vi "PicoScopeospaSettings.vi"(0 "handle in":i16=16384, 1 "Device Info":T3={"PICO_DRIVER_VERSION"="", "PICO_USB_VERSION"="", "PICO_HARDWARE_VERSION"="", "PICO_VARIANT_INFO"="", "PICO_BATCH_AND_SERIAL"="", "PICO_CAL_DATE"="", "PICO_KERNEL_VERSION"="", "PICO_DIGITAL_HARDWARE_VERSION"="", "PICO_ANALOGUE_HARDWARE_VERSION"="", "PICO_FIRMWARE_VERSION_1"="", "PICO_FIRMWARE_VERSION_2"="", "PICO_IPP_VERSION"="", "PICO_DRIVER_PATH"="", "PICO_FIRMWARE_VERSION_3"="", "PICO_FRONT_PANEL_FIRMWARE_VERSION"="", "Number of Channels"=0, "MSO"=TRUE}, 2 "Channels":T2={"Channel A Settings "={"Enabled"=FALSE, "Coupling"=1, "Range"=8, "Analogue Offset"=0.0, "BandWidth"=0, "PROBE_RANGE_INFO"=0}, "Channel B Settings "={"Enabled"=FALSE, "Coupling"=1, "Range"=8, "Analogue Offset"=0.0, "BandWidth"=0, "PROBE_RANGE_INFO"=0}, "Channel C Settings "={"Enabled"=FALSE, "Coupling"=1, "Range"=8, "Analogue Offset"=0.0, "BandWidth"=0, "PROBE_RANGE_INFO"=0}, "Channel D Settings "={"Enabled"=FALSE, "Coupling"=1, "Range"=8, "Analogue Offset"=0.0, "BandWidth"=0, "PROBE_RANGE_INFO"=0}, "Channel E Settings "={"Enabled"=FALSE, "Coupling"=50, "Range"=5, "Analogue Offset"=0.0, "BandWidth"=0, "PROBE_RANGE_INFO"=0}, "Channel F Settings "={"Enabled"=FALSE, "Coupling"=50, "Range"=5, "Analogue Offset"=0.0, "BandWidth"=0, "PROBE_RANGE_INFO"=0}, "Channel G Settings "={"Enabled"=FALSE, "Coupling"=50, "Range"=5, "Analogue Offset"=0.0, "BandWidth"=0, "PROBE_RANGE_INFO"=0}, "Channel H Settings "={"Enabled"=FALSE, "Coupling"=50, "Range"=5, "Analogue Offset"=0.0, "BandWidth"=0, "PROBE_RANGE_INFO"=0}} {"Channel H Settings"."PROBE_RANGE_INFO" items=["PROBE_NONE_NV"=0, "X1_PROBE_NV"=1, "X10_PROBE_NV"=10]; "Channel H Settings"."BandWidth" items=["Full"=0, "100kHz"=100000, "20kHz"=200000, "1MHz"=1000000, "20MHz"=20000000, "25MHz"=25000000, "50MHz"=50000000, "200MHz"=200000000, "250MHz"=250000000, "500MHz"=500000000]; "Channel H Settings"."Range" items=["10mV"=0, "20mV"=1, "50mV"=2, "100mV"=3, "200mV"=4, "500mV"=5, "1V"=6, "2V"=7, "5V"=8, "10V"=9, "20V"=10, "50V"=11, "100V"=12, "200V"=13, "x10_Probe_100mV"=32, "x10_Probe_200mV"=33, "x10_Probe_500mV"=34, "x10_Probe_1V"=35, "x10_Probe_2V"=36, "x10_Probe_5V"=37, "x10_Probe_10V"=38, "x10_Probe_20V"=39, "x10_Probe_50V"=40, "x10_Probe_100V"=41, "x10_Probe_200V"=42, "x10_Probe_500V"=43, "CURRENT_CLAMP_60A_2A"=10500, "CURRENT_CLAMP_60A_5A"=10501, "CURRENT_CLAMP_60A_10A"=10502, "CURRENT_CLAMP_60A_20A"=10503, "CURRENT_CLAMP_60A_50A"=10504, "CURRENT_CLAMP_60A_60A"=10505, "CURRENT_CLAMP_60A_V2_0_5A"=10600, "CURRENT_CLAMP_60A_V2_1A"=10601, "CURRENT_CLAMP_60A_V2_2A"=10602, "CURRENT_CLAMP_60A_V2_5A"=10603, "CURRENT_CLAMP_60A_V2_10A"=10604, "CURRENT_CLAMP_60A_V2_20A"=10605, "CURRENT_CLAMP_60A_V2_50A"=10606, "CURRENT_CLAMP_60A_V2_60A"=10607, "RESISTANCE_LEAD_NEG5_TO_20OHM"=7000, "RESISTANCE_LEAD_NEG50_TO_200OHM"=7001, "RESISTANCE_LEAD_NEG500_TO_2KOHM"=7002, "RESISTANCE_LEAD_NEG5K_TO_20KOHM"=7003, "RESISTANCE_LEAD_NEG50K_TO_LEAD_200KOHM"=7004, "RESISTANCE_LEAD_NEG500K_TO_LEAD_2MOHM"=7005, "RESISTANCE_LEAD_DIODE_TEST"=7006, "HT_NEG3_TO_5KV"=8950, "HT_NEG3_TO_10KV"=8951, "HT_NEG5_TO_20KV"=8952, "HT_NEG5_TO_50KV"=8953, "HT_NEG5_TO_100KV"=8954, "HT_NEG3_TO_5KV_INVERTED"=8955, "HT_NEG3_TO_10KV_INVERTED"=8956, "HT_NEG5_TO_20KV_INVERTED"=8957, "HT_NEG5_TO_50KV_INVERTED"=8958, "HT_NEG5_TO_100KV_INVERTED"=8959, "TEMPERATURE_NEG50_TO_150DEGC"=9000, "PRESSURE_SENSOR_-100k-150k_PASCALS"=9100, "PRESSURE_SENSOR_-100k_TO_400k_PASCALS"=9101, "PRESSURE_SENSOR_-200k_TO_800k_PASCALS"=9102, "PRESSURE_SENSOR_-400k_TO_1600k_PASCALS"=9103, "PRESSURE_SENSOR_-400k_TO_3400k_PASCALS"=9104, "PRESSURE_SENSOR_-150k_TO_1350k_PASCALS"=9105]; "Channel H Settings"."Coupling" items=["AC"=0, "DC 1M Ohm"=1, "DC 50 Ohm"=50]; "Channel G Settings"."PROBE_RANGE_INFO" items=["PROBE_NONE_NV"=0, "X1_PROBE_NV"=1, "X10_PROBE_NV"=10]; "Channel G Settings"."BandWidth" items=["Full"=0, "100kHz"=100000, "20kHz"=200000, "1MHz"=1000000, "20MHz"=20000000, "25MHz"=25000000, "50MHz"=50000000, "200MHz"=200000000, "250MHz"=250000000, "500MHz"=500000000]; "Channel G Settings"."Range" items=["10mV"=0, "20mV"=1, "50mV"=2, "100mV"=3, "200mV"=4, "500mV"=5, "1V"=6, "2V"=7, "5V"=8, "10V"=9, "20V"=10, "50V"=11, "100V"=12, "200V"=13, "x10_Probe_100mV"=32, "x10_Probe_200mV"=33, "x10_Probe_500mV"=34, "x10_Probe_1V"=35, "x10_Probe_2V"=36, "x10_Probe_5V"=37, "x10_Probe_10V"=38, "x10_Probe_20V"=39, "x10_Probe_50V"=40, "x10_Probe_100V"=41, "x10_Probe_200V"=42, "x10_Probe_500V"=43, "CURRENT_CLAMP_60A_2A"=10500, "CURRENT_CLAMP_60A_5A"=10501, "CURRENT_CLAMP_60A_10A"=10502, "CURRENT_CLAMP_60A_20A"=10503, "CURRENT_CLAMP_60A_50A"=10504, "CURRENT_CLAMP_60A_60A"=10505, "CURRENT_CLAMP_60A_V2_0_5A"=10600, "CURRENT_CLAMP_60A_V2_1A"=10601, "CURRENT_CLAMP_60A_V2_2A"=10602, "CURRENT_CLAMP_60A_V2_5A"=10603, "CURRENT_CLAMP_60A_V2_10A"=10604, "CURRENT_CLAMP_60A_V2_20A"=10605, "CURRENT_CLAMP_60A_V2_50A"=10606, "CURRENT_CLAMP_60A_V2_60A"=10607, "RESISTANCE_LEAD_NEG5_TO_20OHM"=7000, "RESISTANCE_LEAD_NEG50_TO_200OHM"=7001, "RESISTANCE_LEAD_NEG500_TO_2KOHM"=7002, "RESISTANCE_LEAD_NEG5K_TO_20KOHM"=7003, "RESISTANCE_LEAD_NEG50K_TO_LEAD_200KOHM"=7004, "RESISTANCE_LEAD_NEG500K_TO_LEAD_2MOHM"=7005, "RESISTANCE_LEAD_DIODE_TEST"=7006, "HT_NEG3_TO_5KV"=8950, "HT_NEG3_TO_10KV"=8951, "HT_NEG5_TO_20KV"=8952, "HT_NEG5_TO_50KV"=8953, "HT_NEG5_TO_100KV"=8954, "HT_NEG3_TO_5KV_INVERTED"=8955, "HT_NEG3_TO_10KV_INVERTED"=8956, "HT_NEG5_TO_20KV_INVERTED"=8957, "HT_NEG5_TO_50KV_INVERTED"=8958, "HT_NEG5_TO_100KV_INVERTED"=8959, "TEMPERATURE_NEG50_TO_150DEGC"=9000, "PRESSURE_SENSOR_-100k-150k_PASCALS"=9100, "PRESSURE_SENSOR_-100k_TO_400k_PASCALS"=9101, "PRESSURE_SENSOR_-200k_TO_800k_PASCALS"=9102, "PRESSURE_SENSOR_-400k_TO_1600k_PASCALS"=9103, "PRESSURE_SENSOR_-400k_TO_3400k_PASCALS"=9104, "PRESSURE_SENSOR_-150k_TO_1350k_PASCALS"=9105]; "Channel G Settings"."Coupling" items=["AC"=0, "DC 1M Ohm"=1, "DC 50 Ohm"=50]; "Channel F Settings"."PROBE_RANGE_INFO" items=["PROBE_NONE_NV"=0, "X1_PROBE_NV"=1, "X10_PROBE_NV"=10]; "Channel F Settings"."BandWidth" items=["Full"=0, "100kHz"=100000, "20kHz"=200000, "1MHz"=1000000, "20MHz"=20000000, "25MHz"=25000000, "50MHz"=50000000, "200MHz"=200000000, "250MHz"=250000000, "500MHz"=500000000]; "Channel F Settings"."Range" items=["10mV"=0, "20mV"=1, "50mV"=2, "100mV"=3, "200mV"=4, "500mV"=5, "1V"=6, "2V"=7, "5V"=8, "10V"=9, "20V"=10, "50V"=11, "100V"=12, "200V"=13, "x10_Probe_100mV"=32, "x10_Probe_200mV"=33, "x10_Probe_500mV"=34, "x10_Probe_1V"=35, "x10_Probe_2V"=36, "x10_Probe_5V"=37, "x10_Probe_10V"=38, "x10_Probe_20V"=39, "x10_Probe_50V"=40, "x10_Probe_100V"=41, "x10_Probe_200V"=42, "x10_Probe_500V"=43, "CURRENT_CLAMP_60A_2A"=10500, "CURRENT_CLAMP_60A_5A"=10501, "CURRENT_CLAMP_60A_10A"=10502, "CURRENT_CLAMP_60A_20A"=10503, "CURRENT_CLAMP_60A_50A"=10504, "CURRENT_CLAMP_60A_60A"=10505, "CURRENT_CLAMP_60A_V2_0_5A"=10600, "CURRENT_CLAMP_60A_V2_1A"=10601, "CURRENT_CLAMP_60A_V2_2A"=10602, "CURRENT_CLAMP_60A_V2_5A"=10603, "CURRENT_CLAMP_60A_V2_10A"=10604, "CURRENT_CLAMP_60A_V2_20A"=10605, "CURRENT_CLAMP_60A_V2_50A"=10606, "CURRENT_CLAMP_60A_V2_60A"=10607, "RESISTANCE_LEAD_NEG5_TO_20OHM"=7000, "RESISTANCE_LEAD_NEG50_TO_200OHM"=7001, "RESISTANCE_LEAD_NEG500_TO_2KOHM"=7002, "RESISTANCE_LEAD_NEG5K_TO_20KOHM"=7003, "RESISTANCE_LEAD_NEG50K_TO_LEAD_200KOHM"=7004, "RESISTANCE_LEAD_NEG500K_TO_LEAD_2MOHM"=7005, "RESISTANCE_LEAD_DIODE_TEST"=7006, "HT_NEG3_TO_5KV"=8950, "HT_NEG3_TO_10KV"=8951, "HT_NEG5_TO_20KV"=8952, "HT_NEG5_TO_50KV"=8953, "HT_NEG5_TO_100KV"=8954, "HT_NEG3_TO_5KV_INVERTED"=8955, "HT_NEG3_TO_10KV_INVERTED"=8956, "HT_NEG5_TO_20KV_INVERTED"=8957, "HT_NEG5_TO_50KV_INVERTED"=8958, "HT_NEG5_TO_100KV_INVERTED"=8959, "TEMPERATURE_NEG50_TO_150DEGC"=9000, "PRESSURE_SENSOR_-100k-150k_PASCALS"=9100, "PRESSURE_SENSOR_-100k_TO_400k_PASCALS"=9101, "PRESSURE_SENSOR_-200k_TO_800k_PASCALS"=9102, "PRESSURE_SENSOR_-400k_TO_1600k_PASCALS"=9103, "PRESSURE_SENSOR_-400k_TO_3400k_PASCALS"=9104, "PRESSURE_SENSOR_-150k_TO_1350k_PASCALS"=9105]; "Channel F Settings"."Coupling" items=["AC"=0, "DC 1M Ohm"=1, "DC 50 Ohm"=50]; "Channel E Settings"."PROBE_RANGE_INFO" items=["PROBE_NONE_NV"=0, "X1_PROBE_NV"=1, "X10_PROBE_NV"=10]; "Channel E Settings"."BandWidth" items=["Full"=0, "100kHz"=100000, "20kHz"=200000, "1MHz"=1000000, "20MHz"=20000000, "25MHz"=25000000, "50MHz"=50000000, "200MHz"=200000000, "250MHz"=250000000, "500MHz"=500000000]; "Channel E Settings"."Range" items=["10mV"=0, "20mV"=1, "50mV"=2, "100mV"=3, "200mV"=4, "500mV"=5, "1V"=6, "2V"=7, "5V"=8, "10V"=9, "20V"=10, "50V"=11, "100V"=12, "200V"=13, "x10_Probe_100mV"=32, "x10_Probe_200mV"=33, "x10_Probe_500mV"=34, "x10_Probe_1V"=35, "x10_Probe_2V"=36, "x10_Probe_5V"=37, "x10_Probe_10V"=38, "x10_Probe_20V"=39, "x10_Probe_50V"=40, "x10_Probe_100V"=41, "x10_Probe_200V"=42, "x10_Probe_500V"=43, "CURRENT_CLAMP_60A_2A"=10500, "CURRENT_CLAMP_60A_5A"=10501, "CURRENT_CLAMP_60A_10A"=10502, "CURRENT_CLAMP_60A_20A"=10503, "CURRENT_CLAMP_60A_50A"=10504, "CURRENT_CLAMP_60A_60A"=10505, "CURRENT_CLAMP_60A_V2_0_5A"=10600, "CURRENT_CLAMP_60A_V2_1A"=10601, "CURRENT_CLAMP_60A_V2_2A"=10602, "CURRENT_CLAMP_60A_V2_5A"=10603, "CURRENT_CLAMP_60A_V2_10A"=10604, "CURRENT_CLAMP_60A_V2_20A"=10605, "CURRENT_CLAMP_60A_V2_50A"=10606, "CURRENT_CLAMP_60A_V2_60A"=10607, "RESISTANCE_LEAD_NEG5_TO_20OHM"=7000, "RESISTANCE_LEAD_NEG50_TO_200OHM"=7001, "RESISTANCE_LEAD_NEG500_TO_2KOHM"=7002, "RESISTANCE_LEAD_NEG5K_TO_20KOHM"=7003, "RESISTANCE_LEAD_NEG50K_TO_LEAD_200KOHM"=7004, "RESISTANCE_LEAD_NEG500K_TO_LEAD_2MOHM"=7005, "RESISTANCE_LEAD_DIODE_TEST"=7006, "HT_NEG3_TO_5KV"=8950, "HT_NEG3_TO_10KV"=8951, "HT_NEG5_TO_20KV"=8952, "HT_NEG5_TO_50KV"=8953, "HT_NEG5_TO_100KV"=8954, "HT_NEG3_TO_5KV_INVERTED"=8955, "HT_NEG3_TO_10KV_INVERTED"=8956, "HT_NEG5_TO_20KV_INVERTED"=8957, "HT_NEG5_TO_50KV_INVERTED"=8958, "HT_NEG5_TO_100KV_INVERTED"=8959, "TEMPERATURE_NEG50_TO_150DEGC"=9000, "PRESSURE_SENSOR_-100k-150k_PASCALS"=9100, "PRESSURE_SENSOR_-100k_TO_400k_PASCALS"=9101, "PRESSURE_SENSOR_-200k_TO_800k_PASCALS"=9102, "PRESSURE_SENSOR_-400k_TO_1600k_PASCALS"=9103, "PRESSURE_SENSOR_-400k_TO_3400k_PASCALS"=9104, "PRESSURE_SENSOR_-150k_TO_1350k_PASCALS"=9105]; "Channel E Settings"."Coupling" items=["AC"=0, "DC 1M Ohm"=1, "DC 50 Ohm"=50]; "Channel D Settings"."BandWidth" items=["Full"=0, "100kHz"=100000, "20kHz"=200000, "1MHz"=1000000, "20MHz"=20000000, "25MHz"=25000000, "50MHz"=50000000, "100MHz"=100000000, "200MHz"=200000000, "250MHz"=250000000, "350MHz"=350000000, "500MHz"=500000000]; "Channel D Settings"."PROBE_RANGE_INFO" items=["PROBE_NONE_NV"=0, "X1_PROBE_NV"=1, "X10_PROBE_NV"=10]; "Channel D Settings"."Range" items=["10mV", "20mV", "50mV", "100mV", "200mV", "500mV", "1V", "2V", "5V", "10V", "20V", "50V", "100V", "200V"]; "Channel D Settings"."Coupling" items=["AC"=0, "DC 1M Ohm"=1, "DC 50 Ohm"=50]; "Channel C Settings"."BandWidth" items=["Full"=0, "100kHz"=100000, "20kHz"=200000, "1MHz"=1000000, "20MHz"=20000000, "25MHz"=25000000, "50MHz"=50000000, "100MHz"=100000000, "200MHz"=200000000, "250MHz"=250000000, "350MHz"=350000000, "500MHz"=500000000]; "Channel C Settings"."PROBE_RANGE_INFO" items=["PROBE_NONE_NV"=0, "X1_PROBE_NV"=1, "X10_PROBE_NV"=10]; "Channel C Settings"."Range" items=["10mV", "20mV", "50mV", "100mV", "200mV", "500mV", "1V", "2V", "5V", "10V", "20V", "50V", "100V", "200V"]; "Channel C Settings"."Coupling" items=["AC"=0, "DC 1M Ohm"=1, "DC 50 Ohm"=50]; "Channel B Settings"."BandWidth" items=["Full"=0, "100kHz"=100000, "20kHz"=200000, "1MHz"=1000000, "20MHz"=20000000, "25MHz"=25000000, "50MHz"=50000000, "100MHz"=100000000, "200MHz"=200000000, "250MHz"=250000000, "350MHz"=350000000, "500MHz"=500000000]; "Channel B Settings"."PROBE_RANGE_INFO" items=["PROBE_NONE_NV"=0, "X1_PROBE_NV"=1, "X10_PROBE_NV"=10]; "Channel B Settings"."Range" items=["10mV", "20mV", "50mV", "100mV", "200mV", "500mV", "1V", "2V", "5V", "10V", "20V", "50V", "100V", "200V"]; "Channel B Settings"."Coupling" items=["AC"=0, "DC 1M Ohm"=1, "DC 50 Ohm"=50]; "Channel A Settings"."PROBE_RANGE_INFO" items=["PROBE_NONE_NV"=0, "X1_PROBE_NV"=1, "X10_PROBE_NV"=10]; "Channel A Settings"."Range" items=["10mV", "20mV", "50mV", "100mV", "200mV", "500mV", "1V", "2V", "5V", "10V", "20V", "50V", "100V", "200V"]; "Channel A Settings"."BandWidth" items=["Full"=0, "100kHz"=100000, "20kHz"=200000, "1MHz"=1000000, "20MHz"=20000000, "25MHz"=25000000, "50MHz"=50000000, "100MHz"=100000000, "200MHz"=200000000, "250MHz"=250000000, "350MHz"=350000000, "500MHz"=500000000]; "Channel A Settings"."Coupling" items=["AC"=0, "DC 1M Ohm"=1, "DC 50 Ohm"=50]}, 7 "Max ADC value":i16=32512, 11 "error in (no error)":errorcluster, 12 "Trigger Settings":T4={"Trigger Enabled"=FALSE, "Trigger Threshold (Volts/Probe Units)"=0.0, "Trigger Direction"=2, "Trigger Delay (samples)"=0, "Auto Trigger Time (us)"=1000000, "Trigger Source"=0} {"Trigger Source" items=["Channel A"=0, "Channel B"=1, "Channel C"=2, "Channel D"=3, "Channel E"=4, "Channel F"=5, "Channel G"=6, "Channel H"=7, "Port 0"=128, "Port 1"=129, "Trigger AUX"=1001]; "Trigger Direction" items=["Above", "Below", "Rising", "Falling", "Rising or Falling"]; "Trigger Threshold (Volts/Probe Units)" format="%#_6p"}, 14 "Digital Channels":T1 {"Port 1 Settings"."Threshold Level (Volts)" format="%#_4p"; "Port 0 Settings"."Threshold Level (Volts)" format="%#_4p"}) -> (3 "Enabled array":i16[](array[numeric])=[1, 0, 0, 0, 0, 0, 0, 0, 0, 0], 4 "handle out":i16=16384, 15 "error out":errorcluster)   [LabVIEW 2024]
doc: "Sets up channels and calls setSimpleTrigger"
uses:
  PicoScopeospaAnalogChannelSettings.ctl
  PicoScopeospaDigitalChannelSettings.ctl
  psospa.dll
panel:
  # "D8-D15"
  # "DO-D7"
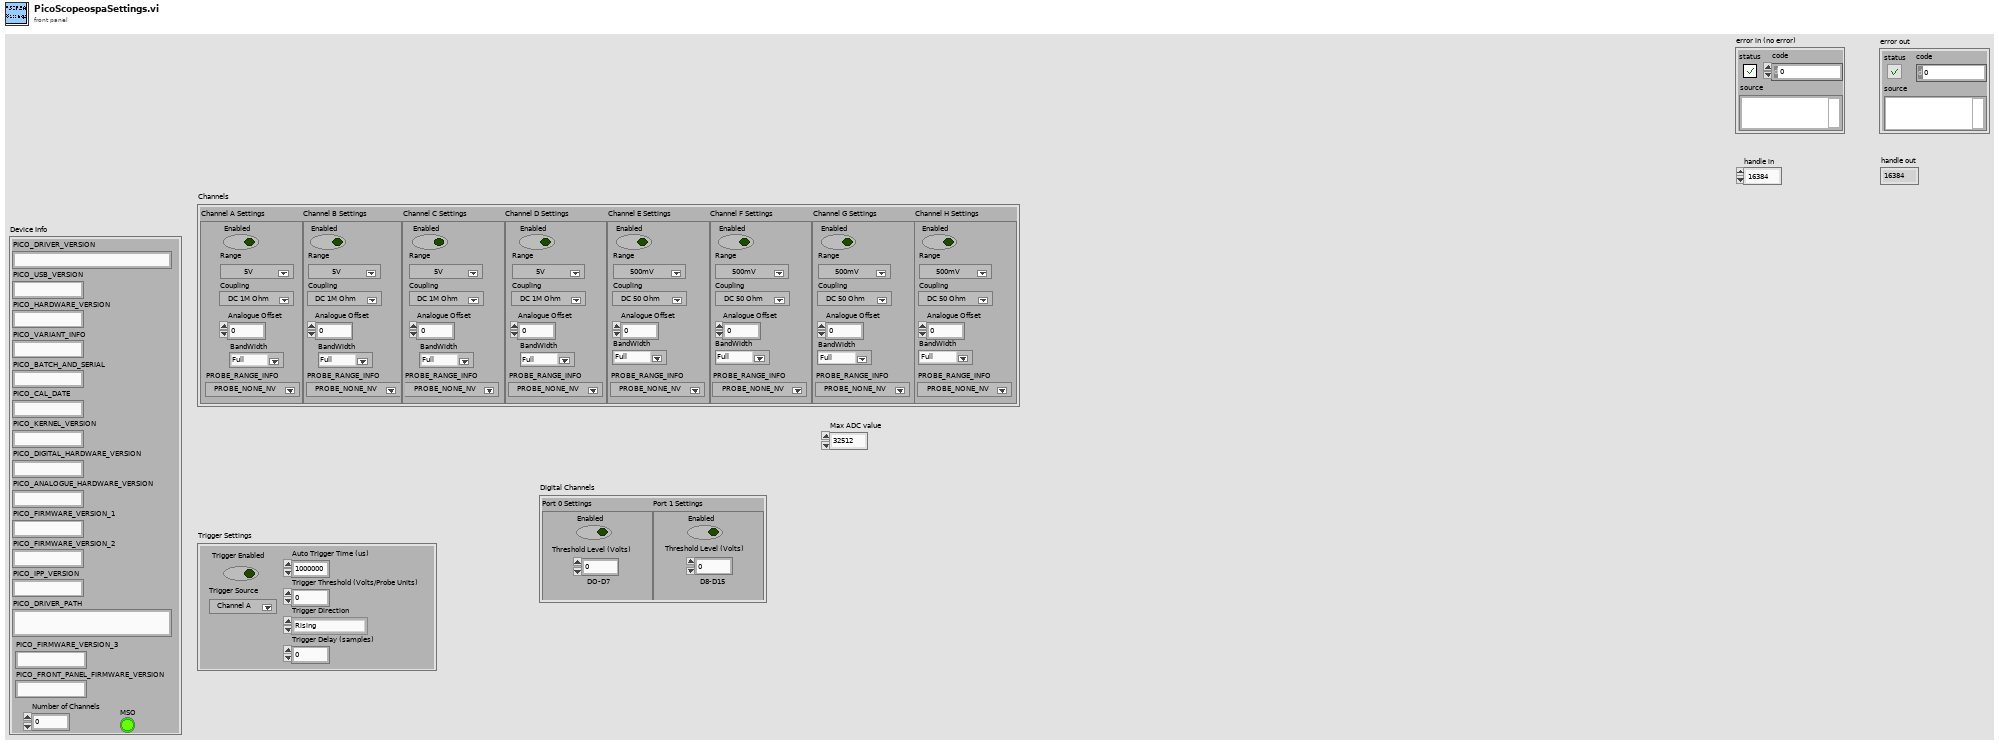
[diagram p1: front panel]
types:
  T1 = typedef "PicoScopeospaDigitalChannelSettings.ctl" = cluster{"Port 0 Settings ":cluster{"Enabled":bool, "Threshold Level (Volts)":dbl}, "Port 1 Settings":cluster{"Enabled":bool, "Threshold Level (Volts)":dbl}}
  T2 = typedef "PicoScopeospaAnalogChannelSettings.ctl" = cluster{"Channel A Settings ":cluster{"Enabled":bool, "Coupling":i16, "Range":u16, "Analogue Offset":dbl, "BandWidth":u32, "PROBE_RANGE_INFO":u32}, "Channel B Settings ":cluster{"Enabled":bool, "Coupling":i16, "Range":u16, "Analogue Offset":dbl, "BandWidth":u32, "PROBE_RANGE_INFO":u32}, "Channel C Settings ":cluster{"Enabled":bool, "Coupling":i16, "Range":u16, "Analogue Offset":dbl, "BandWidth":u32, "PROBE_RANGE_INFO":u32}, "Channel D Settings ":cluster{"Enabled":bool, "Coupling":i16, "Range":u16, "Analogue Offset":dbl, "BandWidth":u32, "PROBE_RANGE_INFO":u32}, "Channel E Settings ":cluster{"Enabled":bool, "Coupling":i16, "Range":u16, "Analogue Offset":dbl, "BandWidth":u32, "PROBE_RANGE_INFO":u32}, "Channel F Settings ":cluster{"Enabled":bool, "Coupling":i16, "Range":u16, "Analogue Offset":dbl, "BandWidth":u32, "PROBE_RANGE_INFO":u32}, "Channel G Settings ":cluster{"Enabled":bool, "Coupling":i16, "Range":u16, "Analogue Offset":dbl, "BandWidth":u32, "PROBE_RANGE_INFO":u32}, "Channel H Settings ":cluster{"Enabled":bool, "Coupling":i16, "Range":u16, "Analogue Offset":dbl, "BandWidth":u32, "PROBE_RANGE_INFO":u32}}
  T3 = cluster{"PICO_DRIVER_VERSION":string, "PICO_USB_VERSION":string, "PICO_HARDWARE_VERSION":string, "PICO_VARIANT_INFO":string, "PICO_BATCH_AND_SERIAL":string, "PICO_CAL_DATE":string, "PICO_KERNEL_VERSION":string, "PICO_DIGITAL_HARDWARE_VERSION":string, "PICO_ANALOGUE_HARDWARE_VERSION":string, "PICO_FIRMWARE_VERSION_1":string, "PICO_FIRMWARE_VERSION_2":string, "PICO_IPP_VERSION":string, "PICO_DRIVER_PATH":string, "PICO_FIRMWARE_VERSION_3":string, "PICO_FRONT_PANEL_FIRMWARE_VERSION":string, "Number of Channels":i16, "MSO":bool}
  T4 = cluster{"Trigger Enabled":bool, "Trigger Threshold (Volts/Probe Units)":dbl, "Trigger Direction":u16, "Trigger Delay (samples)":u64, "Auto Trigger Time (us)":u32, "Trigger Source":u32}
  T5 = cluster{"Enabled":bool, "Coupling":i16, "Range":u16, "Analogue Offset":dbl, "BandWidth":u32, "PROBE_RANGE_INFO":u32}
  T6 = cluster{"status":bool, "code":u32, "source":string}
  T7 = cluster{"Enabled":bool, "Threshold Level (Volts)":dbl}
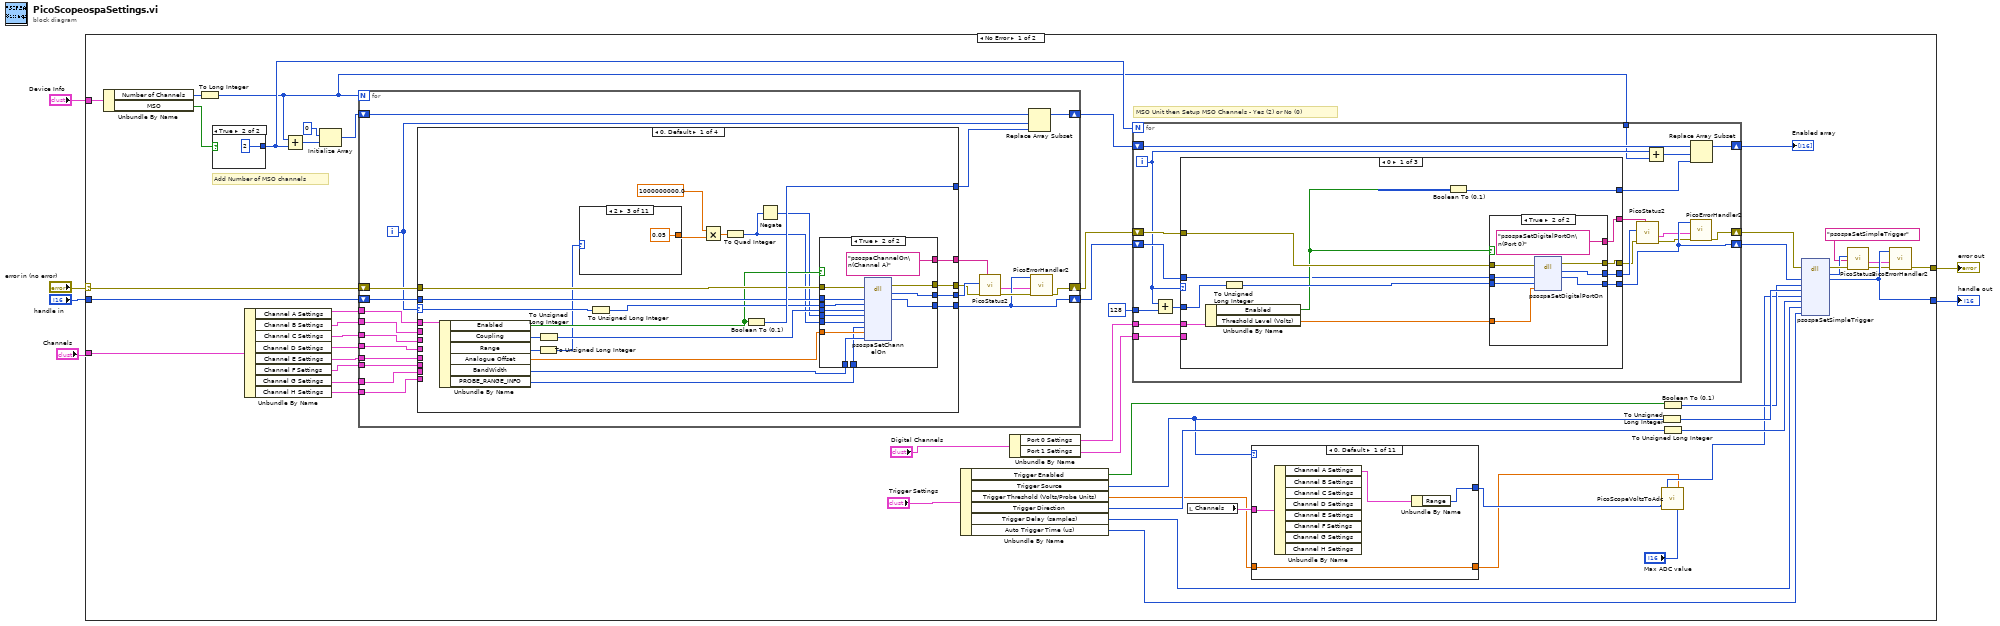
[diagram p0: block diagram]
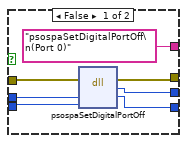
[diagram p2: hidden frame]
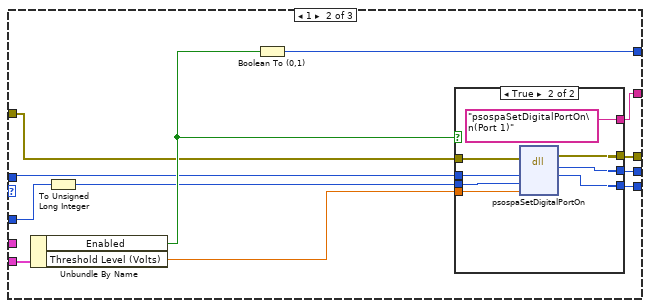
[diagram p3: hidden frame]
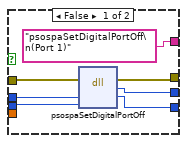
[diagram p4: hidden frame]
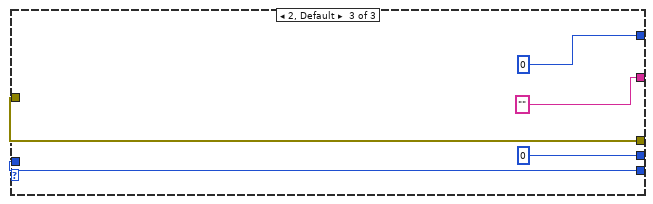
[diagram p5: hidden frame]
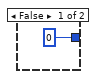
[diagram p6: hidden frame]
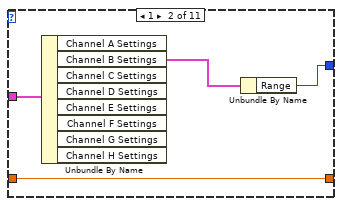
[diagram p7: hidden frame]
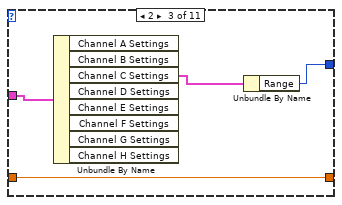
[diagram p8: hidden frame]
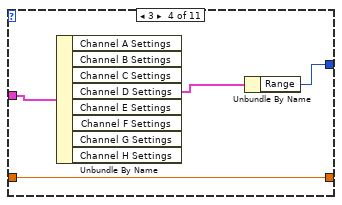
[diagram p9: hidden frame]
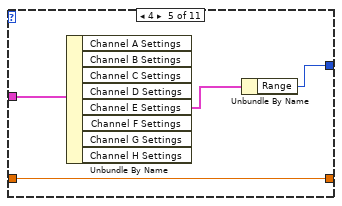
[diagram p10: hidden frame]
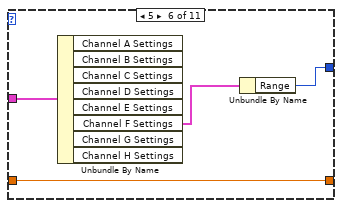
[diagram p11: hidden frame]
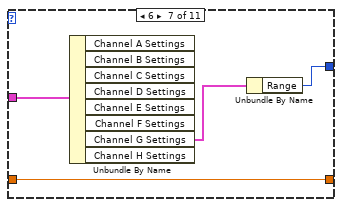
[diagram p12: hidden frame]
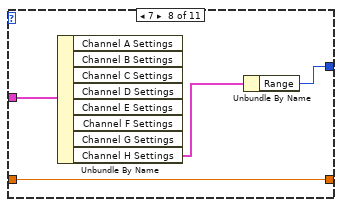
[diagram p13: hidden frame]
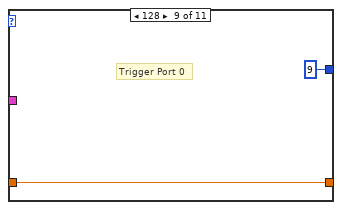
[diagram p14: hidden frame]
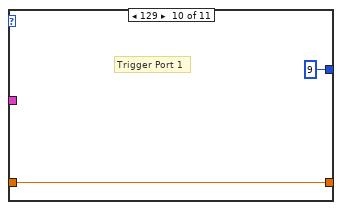
[diagram p15: hidden frame]
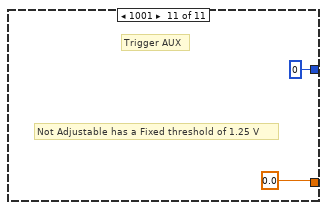
[diagram p16: hidden frame]
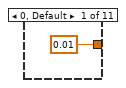
[diagram p17: hidden frame]
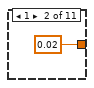
[diagram p18: hidden frame]
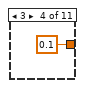
[diagram p19: hidden frame]
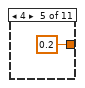
[diagram p20: hidden frame]
diagram:
  n1 = case shown="No Error" "error in (no error)" {
    selector: "error in (no error)" -> [w48 w414]
    tunnel: "handle in" -> [w49 w413]
    tunnel: [w42 w413] -> w6
    tunnel: [w43 w414] -> w5
    tunnel: "Device Info" -> [w45 _]
    tunnel: "Channels" -> [w33 _]
    frame No Error {
      # "Add Number of MSO channels"
      # "MSO Unit then Setup MSO Channels - Yes (2) or No (0)"
      n2 = Unbundle By Name(w45) -> ("Number of Channels"=w44:i16, "MSO"=w16:bool)
      n3 = To Long Integer(number=w44) -> (32bit integer=w13:i32)
      n4 = case shown="True" w16 {
        tunnel: [0 ("y") 2 ("y")] -> w14
        frame False {
        }
        frame True {
        }
      }
      n5 = Unbundle By Name(w33) -> ("Channel A Settings"=w40:T5, "Channel B Settings"=w41:T5, "Channel C Settings"=w39:T5, "Channel D Settings"=w38:T5, "Channel E Settings"=w37:T5, "Channel F Settings"=w34:T5, "Channel G Settings"=w35:T5, "Channel H Settings"=w36:T5)
      n6 = Add(x=w13, y=w14) -> (x+y=w17:i32)
      n7 = Initialize Array(i16 0 ("element"), w17) -> (w46:i16[])
      n8 = for {
        N: w13 -> [_]
        shift-right: [w190] -> w29
        shift-left: w48 -> [w195]
        shift-right: [w185] -> w28
        shift-left: w49 -> [w196]
        shift-right: [w191] -> w31
        shift-left: w46 -> [w192]
        tunnel: w41 -> [w184]
        tunnel: w40 -> [w183]
        tunnel: w39 -> [w182]
        tunnel: w38 -> [w181]
        tunnel: w37 -> [w180]
        tunnel: w36 -> [w179]
        tunnel: w35 -> [w178]
        tunnel: w34 -> [w177]
        i -> [w194]
        n9 = case shown="0, Default" w194 {
          selector: w194 -> [w219 w273 w327 w381]
          tunnel: w196 -> [w212 w266 w320 w374]
          tunnel: w195 -> [w214 w268 w322 w376]
          tunnel: [w216 w270 w324 w378] -> w193
          tunnel: [w207 w261 w315 w369] -> w189
          tunnel: [w213 w267 w321 w375] -> w188
          tunnel: [w215 w269 w323 w377] -> w187
          tunnel: [w206 w260 w314 w368] -> w185
          tunnel: w184 -> [_ w251 _ _]
          tunnel: w183 -> [w205 _ _ _]
          tunnel: w182 -> [_ _ w305 _]
          tunnel: w181 -> [_ _ _ w359]
          tunnel: w180 -> [_ _ _ _]
          tunnel: w179 -> [_ _ _ _]
          tunnel: w178 -> [_ _ _ _]
          tunnel: w177 -> [_ _ _ _]
          frame 0, Default {
            n10 = Unbundle By Name(w205) -> ("Enabled"=w208:bool, "Coupling"=w218:i16, "Range"=w217:u16, "Analogue Offset"=w209:dbl, "BandWidth"=w204:u32, "PROBE_RANGE_INFO"=w200:u32)
            n11 = To Unsigned Long Integer(number=w217) -> (unsigned 32bit integer=w203:u32)
            n12 = To Unsigned Long Integer(number=w218) -> (unsigned 32bit integer=w210:u32)
            n13 = case shown="2" w203 {
              tunnel: [0.01 ("rangeMin") 0.02 ("rangeMin") 0.05 ("rangeMin") 0.1 ("rangeMin") 0.2 ("rangeMin") 0.5 ("rangeMin") 1.0 ("rangeMin") 2.0 ("rangeMin") 5.0 ("rangeMin") 10.0 ("rangeMin") 20.0 ("rangeMin")] -> w202
              frame 0, Default {
              }
              frame 1 {
              }
              frame 2 {
              }
              frame 3 {
              }
              frame 4 {
              }
              frame 5 {
              }
              frame 6 {
              }
              frame 7 {
              }
              frame 8 {
              }
              frame 9 {
              }
              frame 10 {
              }
            }
            n14 = To Unsigned Long Integer(number=w219) -> (unsigned 32bit integer=w211:u32)
            n15 = Multiply(x=1000000000.0, y=w202) -> (x*y=w201:dbl)
            n16 = To Quad Integer(1:w201) -> (0:w198:i64)
            n17 = Boolean To (0,1)(Boolean=w208) -> (0, 1=w216:i16)
            n18 = Negate(x=w198) -> (-x=w199:i64)
            n19 = case shown="True" w208 {
              tunnel: ["psospaSetChannelOff\n(Channel A)" ("source") "psospaChannelOn\n(Channel A)" ("source")] -> w215
              tunnel: w214 -> [w236 w249]
              tunnel: [w235 w248] -> w213
              tunnel: w212 -> [w234 w247]
              tunnel: w211 -> [w233 w246]
              tunnel: w210 -> [_ w245]
              tunnel: w209 -> [_ w244]
              tunnel: [w232 w243] -> w207
              tunnel: [w231 w242] -> w206
              tunnel: w204 -> [_ w241]
              tunnel: w200 -> [_ w240]
              tunnel: w199 -> [_ w238]
              tunnel: w198 -> [_ w239]
              frame False {
                n20 = dll-call lib="F:/Picoscope3000e/Scope_LabView/ps3000e/Treiber_und_SubVis/psospa.dll" fn="psospaSetChannelOff" ("ps3000.dll:_ps3000_open_unit@0")(error in=w236, "handle"=w234, "channel"=w233) -> (error out=w235:errorcluster, "PICO_STATUS"=w232:u32, "handle"=w231:i16)  [unwired: 3 in, 1 out]
              }
              frame True {
                n21 = dll-call lib="F:/Picoscope3000e/Scope_LabView/ps3000e/Treiber_und_SubVis/psospa.dll" fn="psospaSetChannelOn" ("ps3000.dll:_ps3000_open_unit@0")(error in=w249, "handle"=w247, "channel"=w246, "coupling"=w245, "rangeMin"=w238, "rangeMax"=w239, "rangeType"=w240, "analogueOffset"=w244, "bandwidth"=w241) -> (error out=w248:errorcluster, "PICO_STATUS"=w243:u32, "handle"=w242:i16)  [unwired: 9 in, 1 out]
              }
            }
          }
          frame 1 {
            n22 = Unbundle By Name(w251) -> ("Enabled"=w262:bool, "Coupling"=w272:i16, "Range"=w271:u16, "Analogue Offset"=w263:dbl, "BandWidth"=w259:u32, "PROBE_RANGE_INFO"=w255:u32)
            n23 = To Unsigned Long Integer(number=w271) -> (unsigned 32bit integer=w258:u32)
            n24 = To Unsigned Long Integer(number=w272) -> (unsigned 32bit integer=w264:u32)
            n25 = case shown="7" w258 {
              tunnel: [0.01 ("rangeMin") 0.02 ("rangeMin") 0.05 ("rangeMin") 0.1 ("rangeMin") 0.2 ("rangeMin") 0.5 ("rangeMin") 1.0 ("rangeMin") 2.0 ("rangeMin") 5.0 ("rangeMin") 10.0 ("rangeMin") 20.0 ("rangeMin")] -> w257
              frame 0, Default {
              }
              frame 1 {
              }
              frame 2 {
              }
              frame 3 {
              }
              frame 4 {
              }
              frame 5 {
              }
              frame 6 {
              }
              frame 7 {
              }
              frame 8 {
              }
              frame 9 {
              }
              frame 10 {
              }
            }
            n26 = To Unsigned Long Integer(number=w273) -> (unsigned 32bit integer=w265:u32)
            n27 = Multiply(x=1000000000.0, y=w257) -> (x*y=w256:dbl)
            n28 = To Quad Integer(1:w256) -> (0:w253:i64)
            n29 = Boolean To (0,1)(Boolean=w262) -> (0, 1=w270:i16)
            n30 = Negate(x=w253) -> (-x=w254:i64)
            n31 = case shown="False" w262 {
              tunnel: ["psospaSetChannelOff\n(Channel B)" ("source") "psospaChannelOn\n(Channel B)" ("source")] -> w269
              tunnel: w268 -> [w290 w303]
              tunnel: [w289 w302] -> w267
              tunnel: w266 -> [w288 w301]
              tunnel: w265 -> [w287 w300]
              tunnel: w264 -> [_ w299]
              tunnel: w263 -> [_ w298]
              tunnel: [w286 w297] -> w261
              tunnel: [w285 w296] -> w260
              tunnel: w259 -> [_ w295]
              tunnel: w255 -> [_ w294]
              tunnel: w254 -> [_ w292]
              tunnel: w253 -> [_ w293]
              frame False {
                n32 = dll-call lib="F:/Picoscope3000e/Scope_LabView/ps3000e/Treiber_und_SubVis/psospa.dll" fn="psospaSetChannelOff" ("ps3000.dll:_ps3000_open_unit@0")(error in=w290, "handle"=w288, "channel"=w287) -> (error out=w289:errorcluster, "PICO_STATUS"=w286:u32, "handle"=w285:i16)  [unwired: 3 in, 1 out]
              }
              frame True {
                n33 = dll-call lib="F:/Picoscope3000e/Scope_LabView/ps3000e/Treiber_und_SubVis/psospa.dll" fn="psospaSetChannelOn" ("ps3000.dll:_ps3000_open_unit@0")(error in=w303, "handle"=w301, "channel"=w300, "coupling"=w299, "rangeMin"=w292, "rangeMax"=w293, "rangeType"=w294, "analogueOffset"=w298, "bandwidth"=w295) -> (error out=w302:errorcluster, "PICO_STATUS"=w297:u32, "handle"=w296:i16)  [unwired: 9 in, 1 out]
              }
            }
          }
          frame 2 {
            n34 = Unbundle By Name(w305) -> ("Enabled"=w316:bool, "Coupling"=w326:i16, "Range"=w325:u16, "Analogue Offset"=w317:dbl, "BandWidth"=w313:u32, "PROBE_RANGE_INFO"=w309:u32)
            n35 = To Unsigned Long Integer(number=w325) -> (unsigned 32bit integer=w312:u32)
            n36 = To Unsigned Long Integer(number=w326) -> (unsigned 32bit integer=w318:u32)
            n37 = case shown="8" w312 {
              tunnel: [0.01 ("rangeMin") 0.02 ("rangeMin") 0.05 ("rangeMin") 0.1 ("rangeMin") 0.2 ("rangeMin") 0.5 ("rangeMin") 1.0 ("rangeMin") 2.0 ("rangeMin") 5.0 ("rangeMin") 10.0 ("rangeMin") 20.0 ("rangeMin")] -> w311
              frame 0, Default {
              }
              frame 1 {
              }
              frame 2 {
              }
              frame 3 {
              }
              frame 4 {
              }
              frame 5 {
              }
              frame 6 {
              }
              frame 7 {
              }
              frame 8 {
              }
              frame 9 {
              }
              frame 10 {
              }
            }
            n38 = To Unsigned Long Integer(number=w327) -> (unsigned 32bit integer=w319:u32)
            n39 = Multiply(x=1000000000.0, y=w311) -> (x*y=w310:dbl)
            n40 = To Quad Integer(1:w310) -> (0:w307:i64)
            n41 = Boolean To (0,1)(Boolean=w316) -> (0, 1=w324:i16)
            n42 = Negate(x=w307) -> (-x=w308:i64)
            n43 = case shown="True" w316 {
              tunnel: ["psospaSetChannelOff\n(Channel C)" ("source") "psospaChannelOn\n(Channel C)" ("source")] -> w323
              tunnel: w322 -> [w344 w357]
              tunnel: [w343 w356] -> w321
              tunnel: w320 -> [w342 w355]
              tunnel: w319 -> [w341 w354]
              tunnel: w318 -> [_ w353]
              tunnel: w317 -> [_ w352]
              tunnel: [w340 w351] -> w315
              tunnel: [w339 w350] -> w314
              tunnel: w313 -> [_ w349]
              tunnel: w309 -> [_ w348]
              tunnel: w308 -> [_ w346]
              tunnel: w307 -> [_ w347]
              frame False {
                n44 = dll-call lib="F:/Picoscope3000e/Scope_LabView/ps3000e/Treiber_und_SubVis/psospa.dll" fn="psospaSetChannelOff" ("ps3000.dll:_ps3000_open_unit@0")(error in=w344, "handle"=w342, "channel"=w341) -> (error out=w343:errorcluster, "PICO_STATUS"=w340:u32, "handle"=w339:i16)  [unwired: 3 in, 1 out]
              }
              frame True {
                n45 = dll-call lib="F:/Picoscope3000e/Scope_LabView/ps3000e/Treiber_und_SubVis/psospa.dll" fn="psospaSetChannelOn" ("ps3000.dll:_ps3000_open_unit@0")(error in=w357, "handle"=w355, "channel"=w354, "coupling"=w353, "rangeMin"=w346, "rangeMax"=w347, "rangeType"=w348, "analogueOffset"=w352, "bandwidth"=w349) -> (error out=w356:errorcluster, "PICO_STATUS"=w351:u32, "handle"=w350:i16)  [unwired: 9 in, 1 out]
              }
            }
          }
          frame 3 {
            n46 = Unbundle By Name(w359) -> ("Enabled"=w370:bool, "Coupling"=w380:i16, "Range"=w379:u16, "Analogue Offset"=w371:dbl, "BandWidth"=w367:u32, "PROBE_RANGE_INFO"=w363:u32)
            n47 = To Unsigned Long Integer(number=w379) -> (unsigned 32bit integer=w366:u32)
            n48 = To Unsigned Long Integer(number=w380) -> (unsigned 32bit integer=w372:u32)
            n49 = case shown="7" w366 {
              tunnel: [0.01 ("rangeMin") 0.02 ("rangeMin") 0.05 ("rangeMin") 0.1 ("rangeMin") 0.2 ("rangeMin") 0.5 ("rangeMin") 1.0 ("rangeMin") 2.0 ("rangeMin") 5.0 ("rangeMin") 10.0 ("rangeMin") 20.0 ("rangeMin")] -> w365
              frame 0, Default {
              }
              frame 1 {
              }
              frame 2 {
              }
              frame 3 {
              }
              frame 4 {
              }
              frame 5 {
              }
              frame 6 {
              }
              frame 7 {
              }
              frame 8 {
              }
              frame 9 {
              }
              frame 10 {
              }
            }
            n50 = To Unsigned Long Integer(number=w381) -> (unsigned 32bit integer=w373:u32)
            n51 = Multiply(x=1000000000.0, y=w365) -> (x*y=w364:dbl)
            n52 = To Quad Integer(1:w364) -> (0:w361:i64)
            n53 = Boolean To (0,1)(Boolean=w370) -> (0, 1=w378:i16)
            n54 = Negate(x=w361) -> (-x=w362:i64)
            n55 = case shown="True" w370 {
              tunnel: ["psospaSetChannelOff\n(Channel D)" ("source") "psospaChannelOn\n(Channel D)" ("source")] -> w377
              tunnel: w376 -> [w398 w411]
              tunnel: [w397 w410] -> w375
              tunnel: w374 -> [w396 w409]
              tunnel: w373 -> [w395 w408]
              tunnel: w372 -> [_ w407]
              tunnel: w371 -> [_ w406]
              tunnel: [w394 w405] -> w369
              tunnel: [w393 w404] -> w368
              tunnel: w367 -> [_ w403]
              tunnel: w363 -> [_ w402]
              tunnel: w362 -> [_ w400]
              tunnel: w361 -> [_ w401]
              frame False {
                n56 = dll-call lib="F:/Picoscope3000e/Scope_LabView/ps3000e/Treiber_und_SubVis/psospa.dll" fn="psospaSetChannelOff" ("ps3000.dll:_ps3000_open_unit@0")(error in=w398, "handle"=w396, "channel"=w395) -> (error out=w397:errorcluster, "PICO_STATUS"=w394:u32, "handle"=w393:i16)  [unwired: 3 in, 1 out]
              }
              frame True {
                n57 = dll-call lib="F:/Picoscope3000e/Scope_LabView/ps3000e/Treiber_und_SubVis/psospa.dll" fn="psospaSetChannelOn" ("ps3000.dll:_ps3000_open_unit@0")(error in=w411, "handle"=w409, "channel"=w408, "coupling"=w407, "rangeMin"=w400, "rangeMax"=w401, "rangeType"=w402, "analogueOffset"=w406, "bandwidth"=w403) -> (error out=w410:errorcluster, "PICO_STATUS"=w405:u32, "handle"=w404:i16)  [unwired: 9 in, 1 out]
              }
            }
          }
        }
        n58 = call "PicoStatus2.vi"("PICO source"=w187, "Error in"=w188, "PICO STATUS"=w189) -> ("error out"=w186:errorcluster, "PICO_STATUS out"=w176:T6)  [unwired: 5 in]
        n59 = Replace Array Subset(array=w192, new element=w193, index=w194) -> (w191:i16[])
        n60 = call "PicoErrorHandler2.vi"("error in (no error)"=w186, "PICO_STATUS in"=w176, "handle In"=w185) -> ("error out"=w190:errorcluster)  [unwired: 8 in]
      }
      n61 = Unbundle By Name("Trigger Settings") -> ("Trigger Enabled"=w51:bool, "Trigger Source"=w21:u32, "Trigger Threshold (Volts/Probe Units)"=w20:dbl, "Trigger Direction"=w54:u16, "Trigger Delay (samples)"=w53:u64, "Auto Trigger Time (us)"=w52:u32)
      n62 = Unbundle By Name("Digital Channels") -> ("Port 0 Settings"=w30:T7, "Port 1 Settings"=w25:T7)
      n63 = for {
        N: w14 -> [_]
        shift-right: [w71] -> w27
        shift-left: w29 -> [w75]
        shift-right: [w70] -> w26
        shift-left: w28 -> [w76]
        shift-right: [w72] -> w32
        shift-left: w31 -> [w73]
        tunnel: w30 -> [w69]
        tunnel: 128 -> [w67]
        tunnel: w25 -> [w65]
        tunnel: w13 -> [w63]
        i -> [w66]
        n64 = Add(x=w66, y=w67) -> (x+y=w68:i32)
        n65 = case shown="0" w66 {
          tunnel: w76 -> [w82 w106 w134]
          tunnel: w75 -> [w87 w108 w135]
          tunnel: [w88 w115 i16 0] -> w74
          tunnel: [w85 w113 u32 0 ("PICO_STATUS")] -> w60
          tunnel: [w77 w114 w135] -> w59
          tunnel: [w84 w112 w134] -> w70
          tunnel: w69 -> [w80 _ _]
          tunnel: w68 -> [w81 w111 _]
          tunnel: w65 -> [_ w110 _]
          tunnel: [w78 w104 "" ("source")] -> w62
          frame 0 {
            n66 = Unbundle By Name(w80) -> ("Enabled"=w83:bool, "Threshold Level (Volts)"=w79:dbl)
            n67 = To Unsigned Long Integer(number=w81) -> (unsigned 32bit integer=w86:u32)
            n68 = Boolean To (0,1)(Boolean=w83) -> (0, 1=w88:i16)
            n69 = case shown="True" w83 {
              tunnel: ["psospaSetDigitalPortOff\n(Port 0)" ("source") "psospaSetDigitalPortOn\n(Port 0)" ("source")] -> w78
              tunnel: w87 -> [w94 w102]
              tunnel: [w93 w101] -> w77
              tunnel: w86 -> [w92 w100]
              tunnel: [w91 w99] -> w85
              tunnel: [w90 w98] -> w84
              tunnel: w82 -> [w89 w97]
              tunnel: w79 -> [_ w96]
              frame False {
                n70 = dll-call lib="F:/Picoscope3000e/Scope_LabView/ps3000e/Treiber_und_SubVis/psospa.dll" fn="psospaSetDigitalPortOff" ("ps3000.dll:_ps3000_open_unit@0")(error in=w94, "handle"=w89, "port"=w92) -> (error out=w93:errorcluster, "PICO_STATUS"=w91:u32, "handle"=w90:i16)  [unwired: 3 in, 1 out]
              }
              frame True {
                n71 = dll-call lib="F:/Picoscope3000e/Scope_LabView/ps3000e/Treiber_und_SubVis/psospa.dll" fn="psospaSetDigitalPortOn" ("ps3000.dll:_ps3000_open_unit@0")(error in=w102, "handle"=w97, "port"=w100, "logicThresholdLevel"=w96) -> (error out=w101:errorcluster, "PICO_STATUS"=w99:u32, "handle"=w98:i16)  [unwired: 4 in, 1 out]
              }
            }
          }
          frame 1 {
            n72 = Unbundle By Name(w110) -> ("Enabled"=w109:bool, "Threshold Level (Volts)"=w105:dbl)
            n73 = To Unsigned Long Integer(number=w111) -> (unsigned 32bit integer=w107:u32)
            n74 = Boolean To (0,1)(Boolean=w109) -> (0, 1=w115:i16)
            n75 = case shown="True" w109 {
              tunnel: ["psospaSetDigitalPortOff\n(Port 1)" ("source") "psospaSetDigitalPortOn\n(Port 1)" ("source")] -> w104
              tunnel: w108 -> [w121 w129]
              tunnel: [w120 w128] -> w114
              tunnel: w107 -> [w119 w127]
              tunnel: w105 -> [_ w123]
              tunnel: [w118 w126] -> w113
              tunnel: [w117 w125] -> w112
              tunnel: w106 -> [w116 w124]
              frame False {
                n76 = dll-call lib="F:/Picoscope3000e/Scope_LabView/ps3000e/Treiber_und_SubVis/psospa.dll" fn="psospaSetDigitalPortOff" ("ps3000.dll:_ps3000_open_unit@0")(error in=w121, "handle"=w116, "port"=w119) -> (error out=w120:errorcluster, "PICO_STATUS"=w118:u32, "handle"=w117:i16)  [unwired: 3 in, 1 out]
              }
              frame True {
                n77 = dll-call lib="F:/Picoscope3000e/Scope_LabView/ps3000e/Treiber_und_SubVis/psospa.dll" fn="psospaSetDigitalPortOn" ("ps3000.dll:_ps3000_open_unit@0")(error in=w129, "handle"=w124, "port"=w127, "logicThresholdLevel"=w123) -> (error out=w128:errorcluster, "PICO_STATUS"=w126:u32, "handle"=w125:i16)  [unwired: 4 in, 1 out]
              }
            }
          }
          frame 2, Default {
          }
        }
        n78 = call "PicoStatus2.vi"("PICO source"=w62, "Error in"=w59, "PICO STATUS"=w60) -> ("error out"=w58:errorcluster, "PICO_STATUS out"=w61:T6)  [unwired: 5 in]
        n79 = Add(x=w66, y=w63) -> (x+y=w64:i32)
        n80 = call "PicoErrorHandler2.vi"("error in (no error)"=w58, "PICO_STATUS in"=w61, "handle In"=w70) -> ("error out"=w71:errorcluster)  [unwired: 8 in]
        n81 = Replace Array Subset(array=w73, new element=w74, index=w64) -> (w72:i16[])
      }
      "Enabled array" <- w32
      n82 = local read "Channels"() -> (w24:T2)
      n83 = case shown="0, Default" w21 {
        tunnel: [w141 w145 w149 w153 w157 w161 w165 w169 u16 9 ("Range") u16 9 ("Range") u16 0 ("Range")] -> w19
        tunnel: w24 -> [w140 w144 w148 w152 w156 w160 w164 w168 _ _ _]
        tunnel: w20 -> [w138 w142 w146 w150 w154 w158 w162 w166 w170 w172 _]
        tunnel: [w138 w142 w146 w150 w154 w158 w162 w166 w170 w172 0.0 ("Trigger Threshold (Volts/Probe Units)")] -> w18
        frame 0, Default {
          n84 = Unbundle By Name(w140) -> ("Channel A Settings"=w139:T5)  [unwired: 7 out]
          n85 = Unbundle By Name(w139) -> ("Range"=w141:u16)
        }
        frame 1 {
          n86 = Unbundle By Name(w144) -> ("Channel B Settings"=w143:T5)  [unwired: 7 out]
          n87 = Unbundle By Name(w143) -> ("Range"=w145:u16)
        }
        frame 2 {
          n88 = Unbundle By Name(w148) -> ("Channel C Settings"=w147:T5)  [unwired: 7 out]
          n89 = Unbundle By Name(w147) -> ("Range"=w149:u16)
        }
        frame 3 {
          n90 = Unbundle By Name(w152) -> ("Channel D Settings"=w151:T5)  [unwired: 7 out]
          n91 = Unbundle By Name(w151) -> ("Range"=w153:u16)
        }
        frame 4 {
          n92 = Unbundle By Name(w156) -> ("Channel E Settings"=w155:T5)  [unwired: 7 out]
          n93 = Unbundle By Name(w155) -> ("Range"=w157:u16)
        }
        frame 5 {
          n94 = Unbundle By Name(w160) -> ("Channel F Settings"=w159:T5)  [unwired: 7 out]
          n95 = Unbundle By Name(w159) -> ("Range"=w161:u16)
        }
        frame 6 {
          n96 = Unbundle By Name(w164) -> ("Channel G Settings"=w163:T5)  [unwired: 7 out]
          n97 = Unbundle By Name(w163) -> ("Range"=w165:u16)
        }
        frame 7 {
          n98 = Unbundle By Name(w168) -> ("Channel H Settings"=w167:T5)  [unwired: 7 out]
          n99 = Unbundle By Name(w167) -> ("Range"=w169:u16)
        }
        frame 128 {
          # "Trigger Port 0"
        }
        frame 129 {
          # "Trigger Port 1"
        }
        frame 1001 {
          # "Not Adjustable has a Fixed threshold of 1.25 V"
          # "Trigger AUX"
        }
      }
      n100 = To Unsigned Long Integer(number=w21) -> (unsigned 32bit integer=w57:u32)
      n101 = Boolean To (0,1)(Boolean=w51) -> (0, 1=w50:i16)
      n102 = To Unsigned Long Integer(number=w54) -> (unsigned 32bit integer=w56:u32)
      n103 = call "PicoScopeVoltsToAdc.vi"("Max_adc"="Max ADC value", "Units"=w18, "Range Index"=w19) -> ("ADC count"=w22:i16)
      n104 = dll-call lib="F:/Picoscope3000e/Scope_LabView/ps3000e/Treiber_und_SubVis/psospa.dll" fn="psospaSetSimpleTrigger" ("ps3000.dll:_ps3000_open_unit@0")(error in=w27, "handle"=w26, "enable"=w50, "source"=w57, "threshold"=w22, "direction"=w56, "delay"=w53, "autoTrigger_us"=w52) -> (error out=w11:errorcluster, "PICO_STATUS"=w10:u32, "handle"=w42:i16)  [unwired: 8 in, 1 out]
      n105 = call "PicoStatus2.vi"("PICO source"="psospaSetSimpleTrigger" ("source"), "Error in"=w11, "PICO STATUS"=w10) -> ("error out"=w8:errorcluster, "PICO_STATUS out"=w7:T6)  [unwired: 5 in]
      n106 = call "PicoErrorHandler2.vi"("error in (no error)"=w8, "PICO_STATUS in"=w7, "handle In"=w42) -> ("error out"=w43:errorcluster)  [unwired: 8 in]
    }
    frame Error {
    }
  }
  "error out" <- w5
  "handle out" <- w6
